vi "DestroySelfReference.vi"(8 "error in (no error)":errorcluster, 11 "SMO":refnum<class "SMO.lvclass">) -> (0 "error out":errorcluster, 3 "SMO out":refnum<class "SMO.lvclass">)   [LabVIEW 2013, in "SMO.lvclass"]
uses:
  SMO.lvclass
  SMO.lvclass/SMO.ctl
panel:
  # "For instructions on how to use the JKI State Machine Objects, examples and video tutorials, visit:\nhttp://jki.net/state-machine-objects/\n\nJKI State Machine Objects™\nhttp://jki.net/state-machine-objects/\nCopyright (C) 2005-2015, JKI <info@jki.net>\nALL RIGHTS RESERVED"
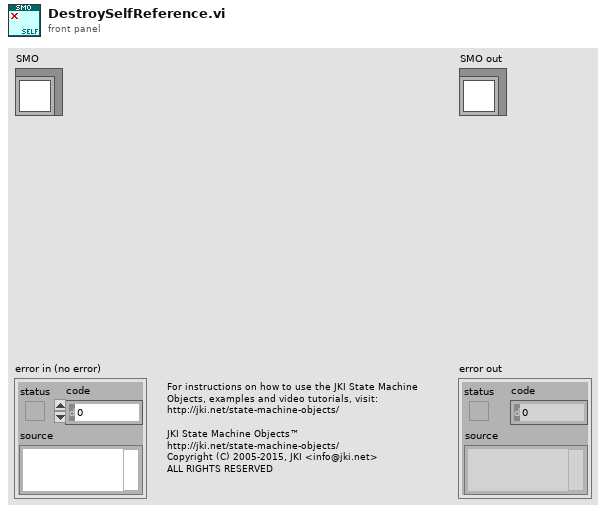
[diagram p1: front panel]
types:
  T1 = typedef "SMO.lvclass/PrivateData--Ref.ctl" = refnum<data-value>
  T2 = typedef "SMO.lvclass/PrivateData--Cluster.ctl" = cluster{"SMO Name":string, "Parent Call":T3, "Registered Processes":T4[], "Process Sync RendezVous":T5, "Process Error Notifier":refnum<notifier>, "Protected Events":T6, "Public Events":T7}
  T3 = typedef "SMO.lvclass/Parent Call--Enum.ctl" = enum16{"Allows parent to run", "Does not request parent to run"}
  T4 = typedef "SMO.lvclass/RegisteredProcessData--Cluster.ctl" = cluster{"Name":string, "Static VI Ref":refnum<vi>, "Running":bool}
  T5 = typedef "Rendezvous RefNum" = refnum<k1>
  T6 = typedef "SMO.lvclass/Protected Events.ctl" = cluster{"StopProcesses":refnum<user-event>, "AbortProcesses":refnum<user-event>}
  T7 = typedef "SMO.lvclass/Public Events.ctl" = cluster{"Error":refnum<user-event>}
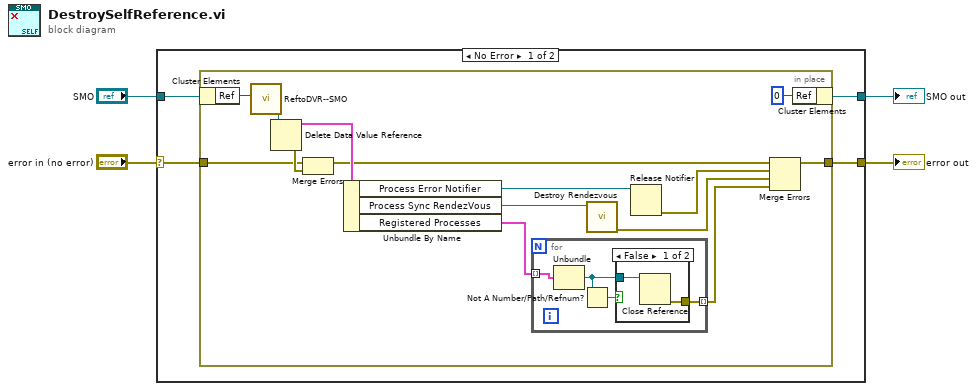
[diagram p0: block diagram]
diagram:
  n1 = case shown="No Error" "error in (no error)" {
    selector: "error in (no error)" -> [w8 w30]
    tunnel: [w7 w30] -> w3
    tunnel: [w5 w29] -> w1
    tunnel: "SMO" -> [w6 w29]
    frame No Error {
      n2 = in-place {
        in-place-border: w8 -> [w13]
        in-place-border: [w22] -> w7
        n3 = in-place-cluster #1(w6) -> ("Ref"=w10:u32)
        n4 = call "ReftoDVR--SMO.vi"("Ref"=w10) -> ("Ref"=w9:T1)  [unwired: 10 in]
        n5 = Delete Data Value Reference(data value reference=w9) -> (data value=w18:T2, error out=w14:errorcluster)  [unwired: 1 in]
        n6 = Merge Errors(w13, w14) -> (w12:errorcluster)
        n7 = Unbundle By Name(w18) -> ("Process Error Notifier"=w19:refnum<notifier>, "Process Sync RendezVous"=w21:T5, "Registered Processes"=w20:T4[])
        n8 = for {
          tunnel: w20 -> [w25] mode=indexing
          tunnel: [w23] -> w15 mode=indexing
          n9 = Unbundle(w25) -> ("Static VI Ref"=w24:refnum<vi>)  [unwired: 2 out]
          n10 = Not A Number/Path/Refnum?(number/path/refnum=w24) -> (NaN/Path/Refnum?=w26:bool)
          n11 = case shown="False" w26 {
            tunnel: w24 -> [w28 _]
            tunnel: [w27 _] -> w23
            frame False {
              n12 = Close Reference(reference=w28) -> (error out=w27:errorcluster)  [unwired: 1 in]
            }
            frame True {
            }
          }
        }
        n13 = call <vilib>:"Destroy Rendezvous.vi"("rendezvous"=w21) -> ("error out"=w16:errorcluster)  [unwired: 5 in, 1 out]
        n14 = Release Notifier(notifier=w19) -> (error out=w17:errorcluster)  [unwired: 2 in, 2 out]
        n15 = Merge Errors(w12, w17, w16, w15) -> (w22:errorcluster)
        n16 = in-place-cluster #1("Ref"=u32 0) -> (w5:refnum<class "SMO.lvclass">)
      }
    }
    frame Error {
    }
  }
  "error out" <- w3
  "SMO out" <- w1
